vi "Lockin.DAQ.Create.AI Task.vi"(8 "error in (no error)":errorcluster, 11 "Lockin.DAQ":refnum<class "Lockin.DAQ.lvclass">) -> (0 "error out":errorcluster, 3 "Lockin.DAQ":refnum<class "Lockin.DAQ.lvclass">)   [LabVIEW 2016, in "Lockin.DAQ.lvclass"]
uses:
  Lockin.DAQ.lvclass
  Lockin.DAQ.lvclass/Lockin.DAQ.ctl
  <vilib>/DAQmx/create/channels.llb/DAQmx Create Channel (AI-Voltage-Basic).vi
  <resource>/objmgr/daqmx.rc
panel:
  out "Current Size":i32
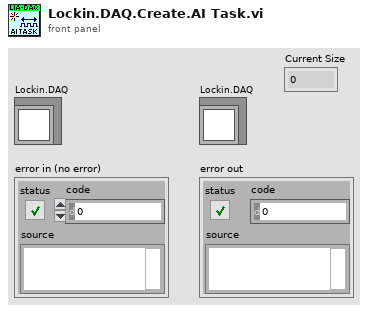
[diagram p1: front panel]
types:
  T1 = typedef "Lockin.DAQ.lvclass/AI.config-array.ctl" = T2[]
  T2 = typedef "Lockin.DAQ.lvclass/AI.config-cluster.ctl" = cluster{"AI.channels":tag, "AI.Coupling":T3, "AI.Range":T4, "input terminal configuration":i32, "DAQ Type":T5}
  T3 = typedef "Lockin.DAQ.lvclass/AI.coupling-enum.ctl" = u16
  T4 = typedef "Lockin.DAQ.lvclass/446xAI-enum.ctl" = enum16{"±0.316", "±1.00", "±3.16", "±10.0", "±31.6", "±42.4"}
  T5 = typedef "Lockin.DAQ.lvclass/DAQType-enum.ctl" = enum16{"None", "USB 4431", "PXI 446x"}
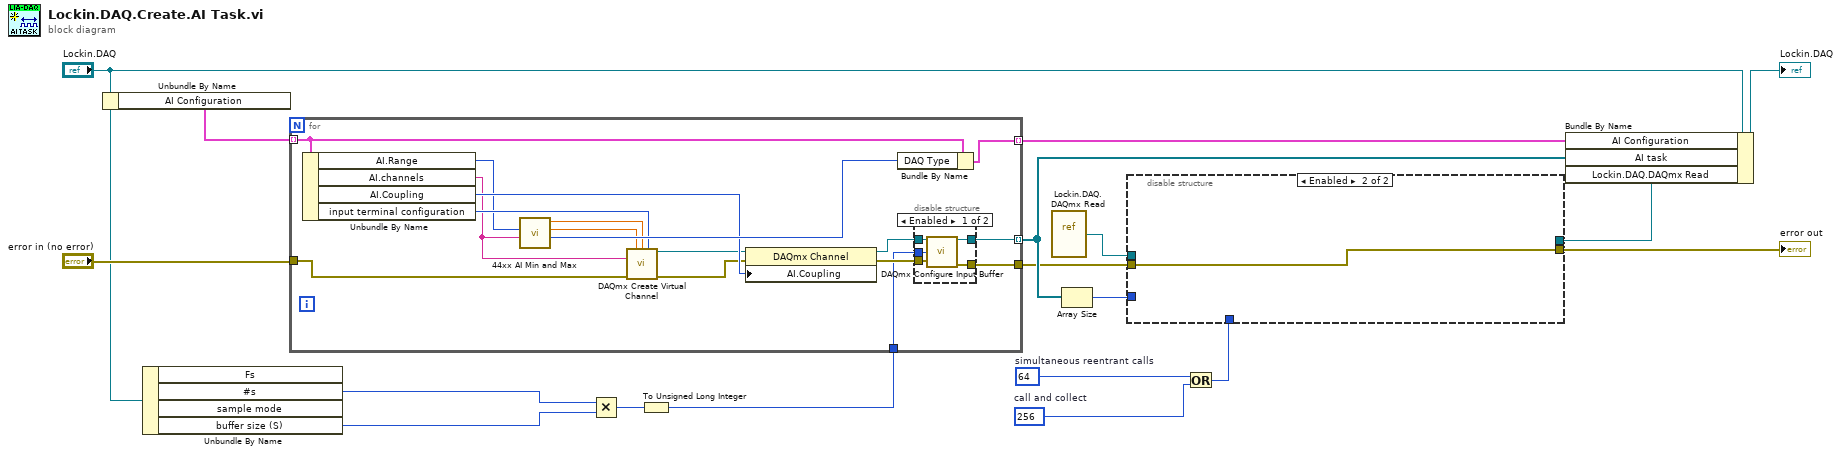
[diagram p0: block diagram]
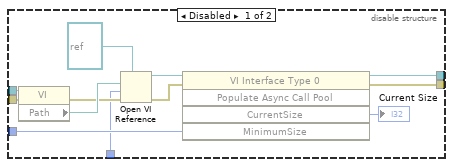
[diagram p2: hidden frame]
diagram:
  w2 = 64  # simultaneous reentrant calls
  w3 = 256  # call and collect
  n1 = Unbundle By Name("Lockin.DAQ") -> ("AI Configuration"=w8:T1)
  n2 = Unbundle By Name("Lockin.DAQ") -> ("#s"=w15:i32, "buffer size (S)"=w14:u32)  [unwired: 2 out]
  n3 = Multiply(x=w15, y=w14) -> (x*y=w16:u32)
  n4 = To Unsigned Long Integer(number=w16) -> (unsigned 32bit integer=w13:u32)
  n5 = for {
    tunnel: [w21] -> w12 mode=indexing
    tunnel: w8 -> [w26] mode=indexing
    tunnel: "error in (no error)" -> [w27]
    tunnel: [w24] -> w7
    tunnel: w13 -> [w22]
    tunnel: [w20] -> w11 mode=indexing
    n6 = Unbundle By Name(w26) -> ("AI.Range"=w32:T4, "AI.channels"=w19:tag, "AI.Coupling"=w33:T3, "input terminal configuration"=w34:i32)
    n7 = call "44xx AI Min and Max.vi"("AI.channels"=w19, "446x AI"=w32) -> ("DAQ Type"=w35:T5, "AI.Max"=w30:dbl, "AI.Min"=w31:dbl)  [unwired: 7 in]
    n8 = call-poly <vilib>:"DAQmx Create Virtual Channel.vi"("maximum value"=w30, "minimum value"=w31, "input terminal configuration"=w34, "physical channels"=w19, "error in"=w27) -> ("task out"=w28:refnum<k21>, "error out"=w29:errorcluster)  [unwired: 9 in]
    n9 = property class="DAQmx Channel"(reference=w28, error in=w29, "AI.Coupling"=w33) -> (reference out=w23:refnum<k21>, error out=w25:errorcluster)
    n10 = Bundle By Name(cluster=w26, "DAQ Type"=w35) -> (w21:T2)
    n11 = disable-structure shown="Enabled" {
      disable-tunnel: w25 -> [w40 w41]
      disable-tunnel: [w39 w41] -> w24
      disable-tunnel: w23 -> [w38 w42]
      disable-tunnel: w22 -> [w37 _]
      disable-tunnel: [w36 w42] -> w20
      frame Enabled {
        n12 = call <vilib>:"DAQmx Configure Input Buffer.vi"("task/channels in"=w38, "buffer size (in samples per channel)"=w37, "error in"=w40) -> ("task out"=w36:refnum<k21>, "error out"=w39:errorcluster)  [unwired: 11 in]
      }
      frame Disabled {
      }
    }
  }
  n13 = vi-ref "Lockin.DAQ.DAQmx Read.vi"() -> (w4:refnum<vi>)
  n14 = Array Size(array=w11) -> (size(s)=w10:i32)
  n15 = Or(x=w2, y=w3) -> (x .or. y?=w1:i32)
  n16 = disable-structure shown="Enabled" {
    disable-tunnel: w10 -> [w49 _]
    disable-tunnel: w7 -> [w48 w55]
    disable-tunnel: [w47 w55] -> w6
    disable-tunnel: [w46 _] -> w5
    disable-tunnel: w4 -> [w45 _]
    disable-tunnel: w1 -> [w43 _]
    frame Disabled {
      n17 = property class="VI"(reference=w45, error in=w48) -> (error out=w53:errorcluster, "Path"=w54:path)  [unwired: 1 out]
      n18 = Open VI Reference(type specifier VI Refnum (for type only)=refnum<vi> refnum, vi path=w54, options=w43, error in (no error)=w53) -> (vi reference=w51:refnum<vi>, error out=w50:errorcluster)  [unwired: 2 in]
      n19 = invoke class="VI Interface Type 0" method="Populate Async Call Pool"(reference=w51, error in=w50, "MinimumSize"=w49) -> (reference out=w46:refnum<vi>, error out=w47:errorcluster, "CurrentSize"=→"Current Size":i32)  [unwired: 2 in, 2 out]
    }
    frame Enabled {
    }
  }
  "error out" <- w6
  n20 = Bundle By Name(cluster="Lockin.DAQ", "AI Configuration"=w12, "AI task"=w11, "Lockin.DAQ.DAQmx Read"=w5) -> (→"Lockin.DAQ":refnum<class "Lockin.DAQ.lvclass">)
